vi "Number of Sample Sets.vi"(11 "Sample Set":dbl[][](array[numeric])) -> (2 "Number of Sample Sets":i32)   [LabVIEW 2011]
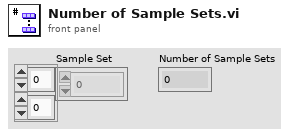
[diagram p1: front panel]
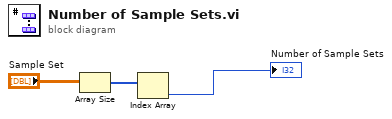
[diagram p0: block diagram]
diagram:
  n1 = Array Size(array="Sample Set") -> (size(s)=w1:i32[])
  n2 = Index Array "Index Array"(array=w1) -> (element=→"Number of Sample Sets":i32)  [unwired: 1 in]
